vi "calcolo rendimento.vi"(0 "Array prove":refnum<vi>[](array[refnum]), 1 "DETERMINAZIONE DEL RENDIMENTO Item Names":string[][](array[string]), 2 "Dati prove":T1, 3 "TABELLE":i16[](array[numeric]), 5 "error in":errorcluster) -> (9 "Eq termico ko":bool, 10 "Coeff correlaz":dbl, 11 "Resistenze ko":bool, 14 "ripeti prova?":bool, 15 "DETERMINAZIONE DEL RENDIMENTO":string[][](array[string]), 16 "Perdite da termica":T6, 17 "Perdite da prova a vuoto 2":T2, 18 "Calcoli da step carichi":T5, 19 "error out":errorcluster)   [LabVIEW 2019]
uses:
  TypeDef/Dati collaudo.ctl
panel:
  in  "Tab Control":T3(tab)
  out "Tabella prova a freddo":i32(listbox)
  in  "Tab Control 3":enum32{"TABELLA ACQUISIZIONI", "Resistenze"}(tab)
  out "Tabella prova a vuoto":i32(listbox)
  out "Resistenze iniziali a vuoto":i32(listbox)
  out "Resistenze finali a vuoto":i32(listbox)
  in  "Tab Control 5":enum32{"TABELLA ACQUISIZIONI", "Resistenze"}(tab)
  out "Tabella prova a carico":i32(listbox)
  out "resistenze iniz a carico":i32(listbox) caption="Resistenze iniziali"
  out "resistenze fin a carico":i32(listbox) caption="Resistenze finali"
  in  "Tab Control 6":T4(tab)
  out "Tabella a freddo - termica":i32(listbox) caption="Tabella misura resistenze a freddo"
  out "Tabella riscaldamento termica":i32(listbox)
  out "Dati riscaldamento":i32(listbox)
  out "Tabella prova a rot blocc":i32(listbox)
  out "Tabella prova coppia max dati":i32(listbox)
  out "Tabella riga coppia max":i32(listbox)
  out "Tabella prova caratt mecc":i32(listbox)
  out "DETERMINAZIONE DEL RENDIMENTO":i32[](listbox)
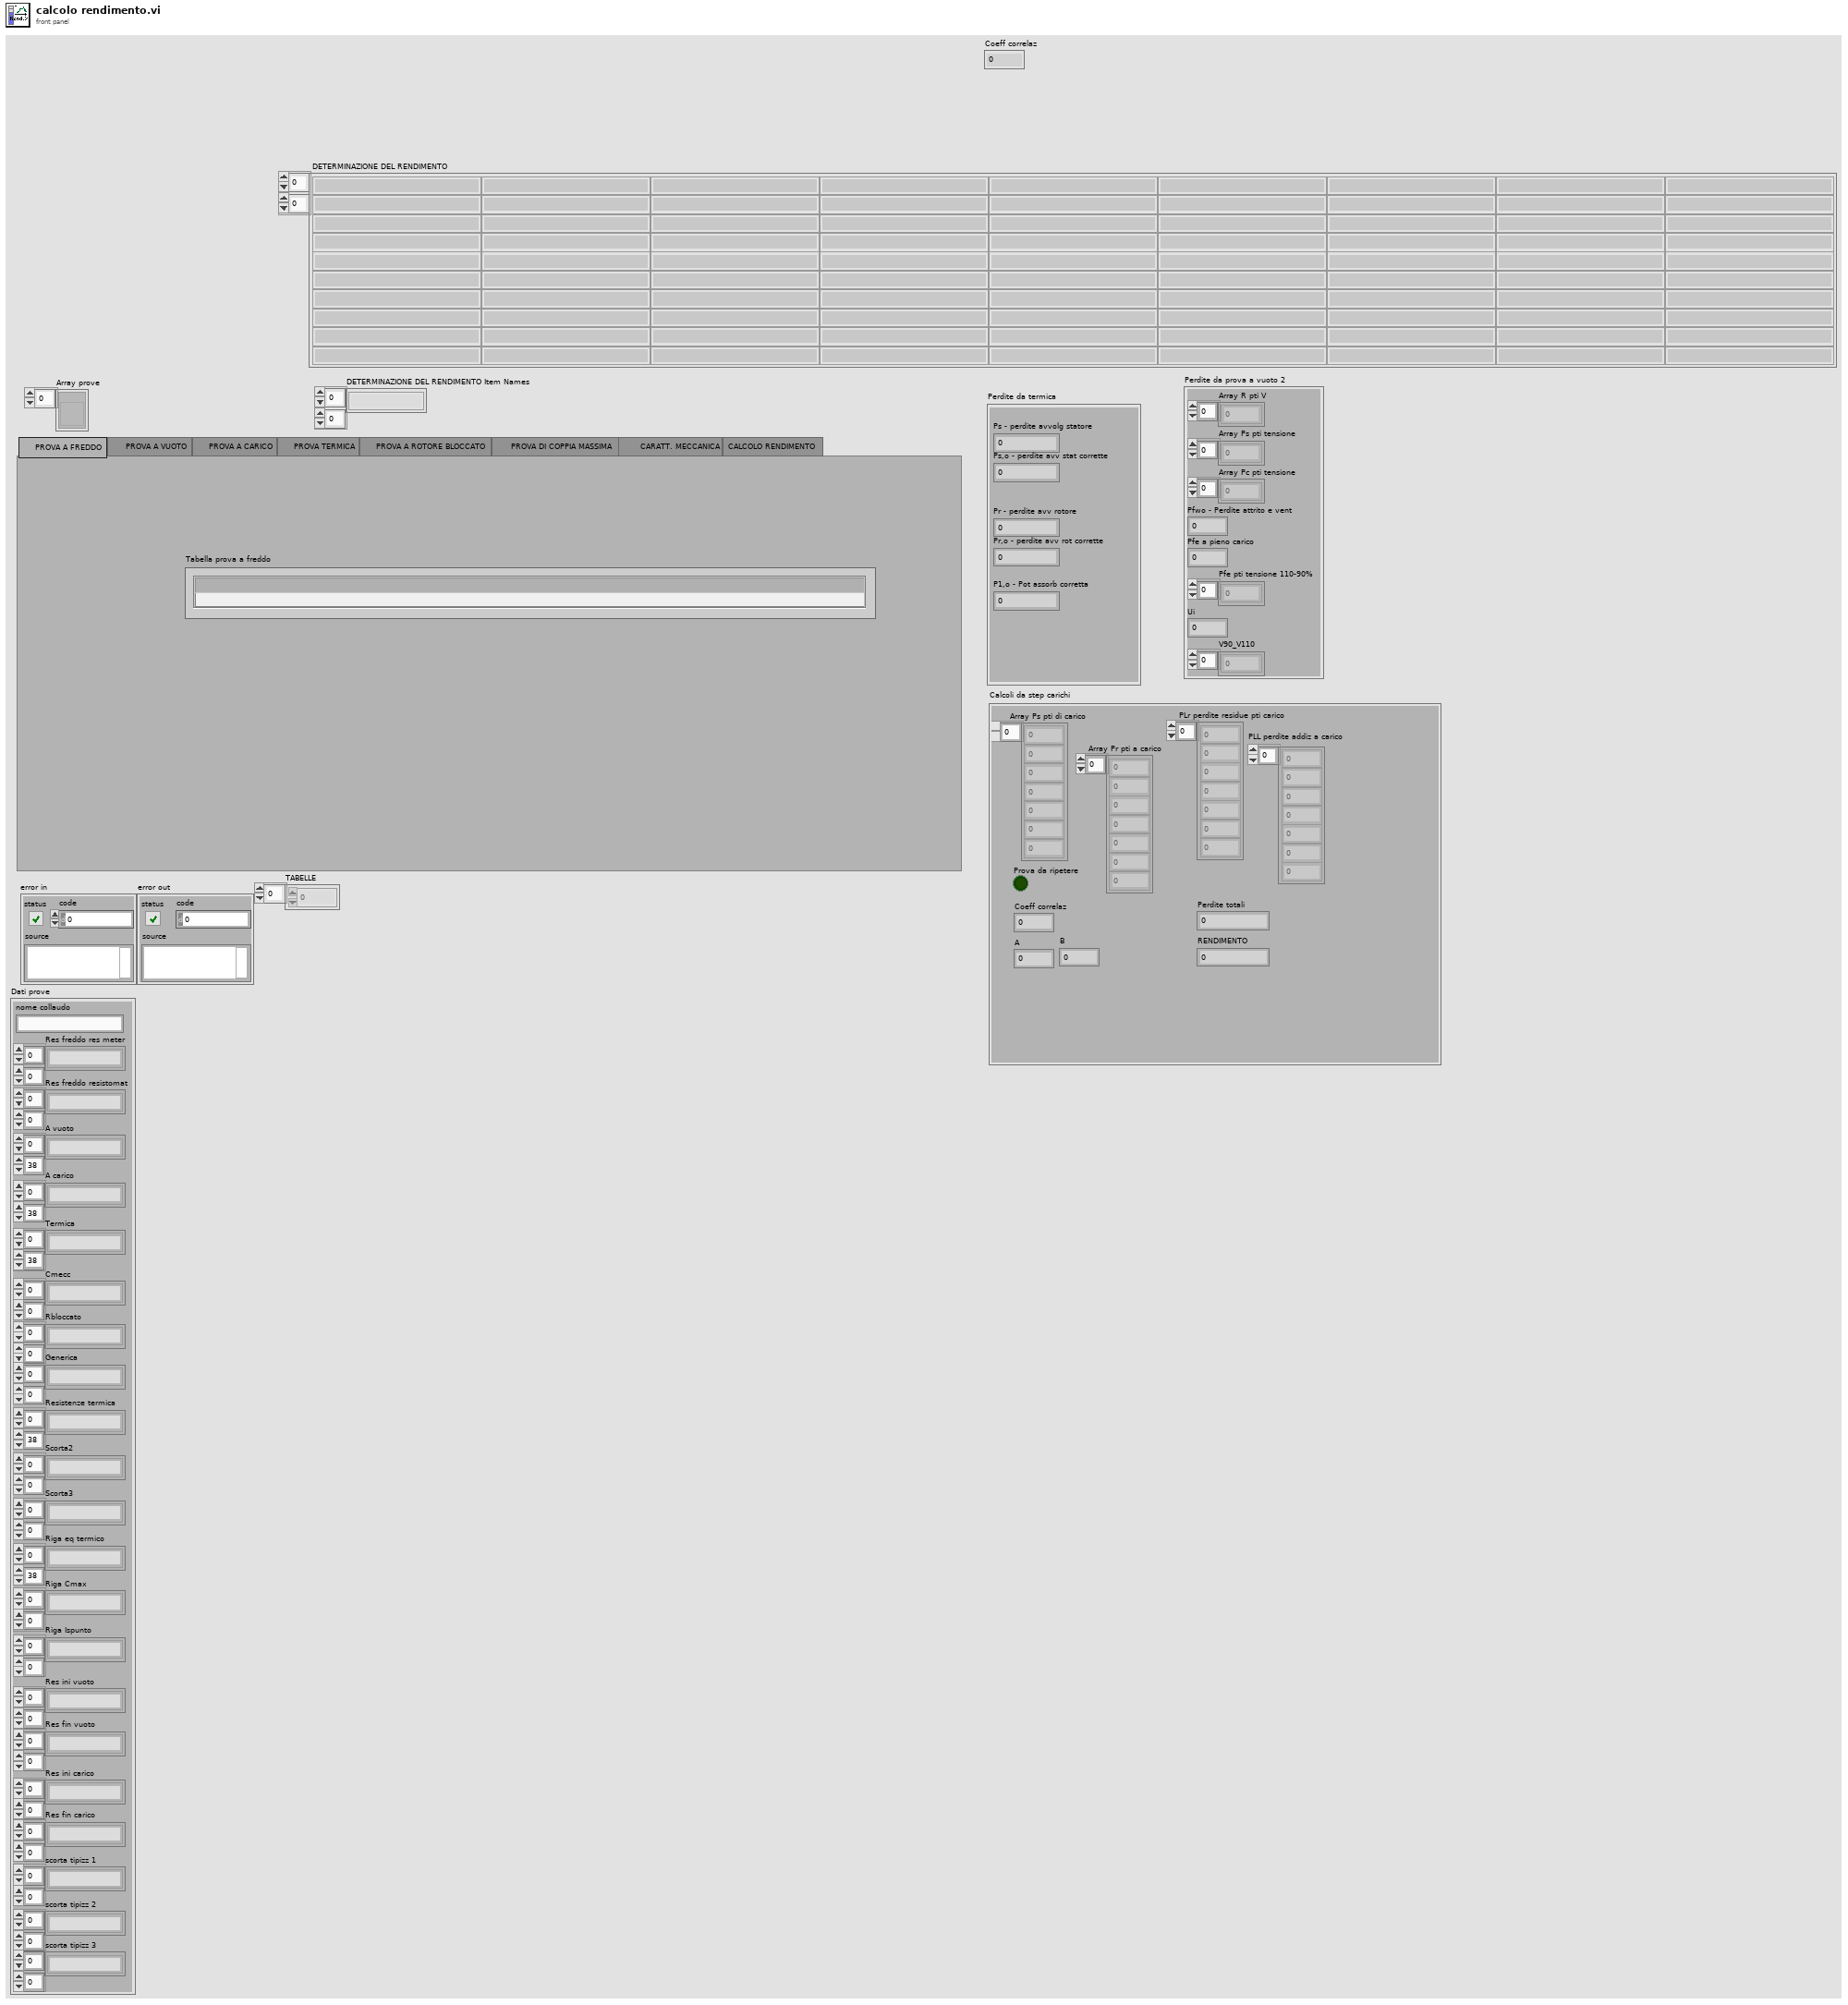
[diagram p1: front panel]
types:
  T1 = typedef "Dati collaudo.ctl" = cluster{"nome collaudo":string, "Res freddo res meter":string[][], "Res freddo resistomat":string[][], "A vuoto":string[][], "A carico":string[][], "Termica":string[][], "Cmecc":string[][], "Rbloccato":string[][], "Generica":string[][], "Resistenze termica":string[][], "Scorta2":string[][], "Scorta3":string[][], "Riga eq termico":string[][], "Riga Cmax":string[][], "Riga Ispunto":string[][], "Res ini vuoto":string[][], "Res fin vuoto":string[][], "Res ini carico":string[][], "Res fin carico":string[][], "scorta tipizz 1":string[][], "scorta tipizz 2":string[][], "scorta tipizz 3":string[][]}
  T2 = cluster{"Array R pti V":dbl[], "Array Ps pti tensione":dbl[], "Array Pc pti tensione":dbl[], "Pfwo - Perdite attrito e vent":dbl, "Pfe a pieno carico":dbl, "Pfe pti tensione 110-90% ":dbl[], "Ui":dbl, "V90_V110":dbl[]}
  T3 = enum32{"    PROVA A FREDDO", "     PROVA A VUOTO", "    PROVA A CARICO", "    PROVA TERMICA", "    PROVA A ROTORE BLOCCATO", "     PROVA DI COPPIA MASSIMA", "      CARATT. MECCANICA", "CALCOLO RENDIMENTO"}
  T4 = enum32{"DATI A FREDDO", "TABELLA ACQ. RISCALDAMENTO", "TABELLA DATI RESISTENZE - DELTA T"}
  T5 = cluster{"Array Ps pti di carico":dbl[], "Array Pr pti a carico":dbl[], "PLr perdite residue pti carico":dbl[], "A":dbl, "B":dbl, "Coeff correlaz":dbl, "Prova da ripetere":bool, "PLL perdite addiz a carico":dbl[], "Perdite totali":dbl, "RENDIMENTO":dbl}
  T6 = cluster{"Ps - perdite avvolg statore":dbl, "Ps,o - perdite avv stat corrette":dbl, "Pr - perdite avv rotore":dbl, "Pr,o - perdite avv rot corrette":dbl, "P1,o - Pot assorb corretta":dbl}
  T7 = cluster{"INDEX R eq termico":i32, "index Tamb caldo":i32, "index dt":i32}
  T8 = cluster{"INDEX P1":i32, "INDEX COPPIA":i32, "INDEX I":i32, "INDEX V":i32, "INDEX SCORR":i32, "INDEX t fluido ingresso":i32, "INDEX P resa":i32, "INDEX tempo":i32, "INDEX dt":i32}
  T9 = cluster{"INDEX P1 W":i32, "INDEX COPPIA":i32, "INDEX I":i32, "INDEX V":i32, "INDEX SCORR":i32, "INDEX t fluido ingresso":i32, "INDEX P resa W":i32, "INDEX tempo s":i32, "INDEX dt":i32}
  T10 = cluster{"INDEX P1":i32, "INDEX COPPIA":i32, "INDEX I":i32, "INDEX V":i32, "INDEX SCORR":i32, "INDEX t fluido ingresso":i32, "INDEX P resa":i32, "INDEX tempo":i32, "INDEX dt":i32}[]
  T11 = cluster{"INDEX R eq termico":i32, "index Tamb caldo":i32, "index dt":i32}[]
  T12 = cluster{"R iniz carico":dbl, "R fin carico":dbl, "Array V carico":dbl[], "Array I carico":dbl[], "Array P elett carico":dbl[], "Array Scorr carico":dbl[], "Array Presa carico":dbl[], "Array Coppia carico":dbl[]}
  T13 = cluster{"R iniz vuoto":dbl, "R fin vuoto":dbl, "Array V0 a vuoto":dbl[], "Array I0 a vuoto":dbl[], "Array P0 a vuoto":dbl[], "Array Scorr a vuoto":dbl[]}
  T14 = cluster{"P1elettrica":dbl, "Coppia":dbl, "I corrente":dbl, "U tensione":dbl, "RPM":dbl, "Freq":dbl, "R eq termico":dbl, "Scorrimento":dbl}
  T15 = cluster{"Rendimenti % a carico":dbl[], "P1 corretta":dbl[], "Scorr corretto":dbl[], "Perdite nel ferro":dbl[], "Perdite mecc corrette":dbl[], "Perdite addiz":dbl[], "perdite statore corrette":dbl[], "perdite rotore corrette":dbl[]}
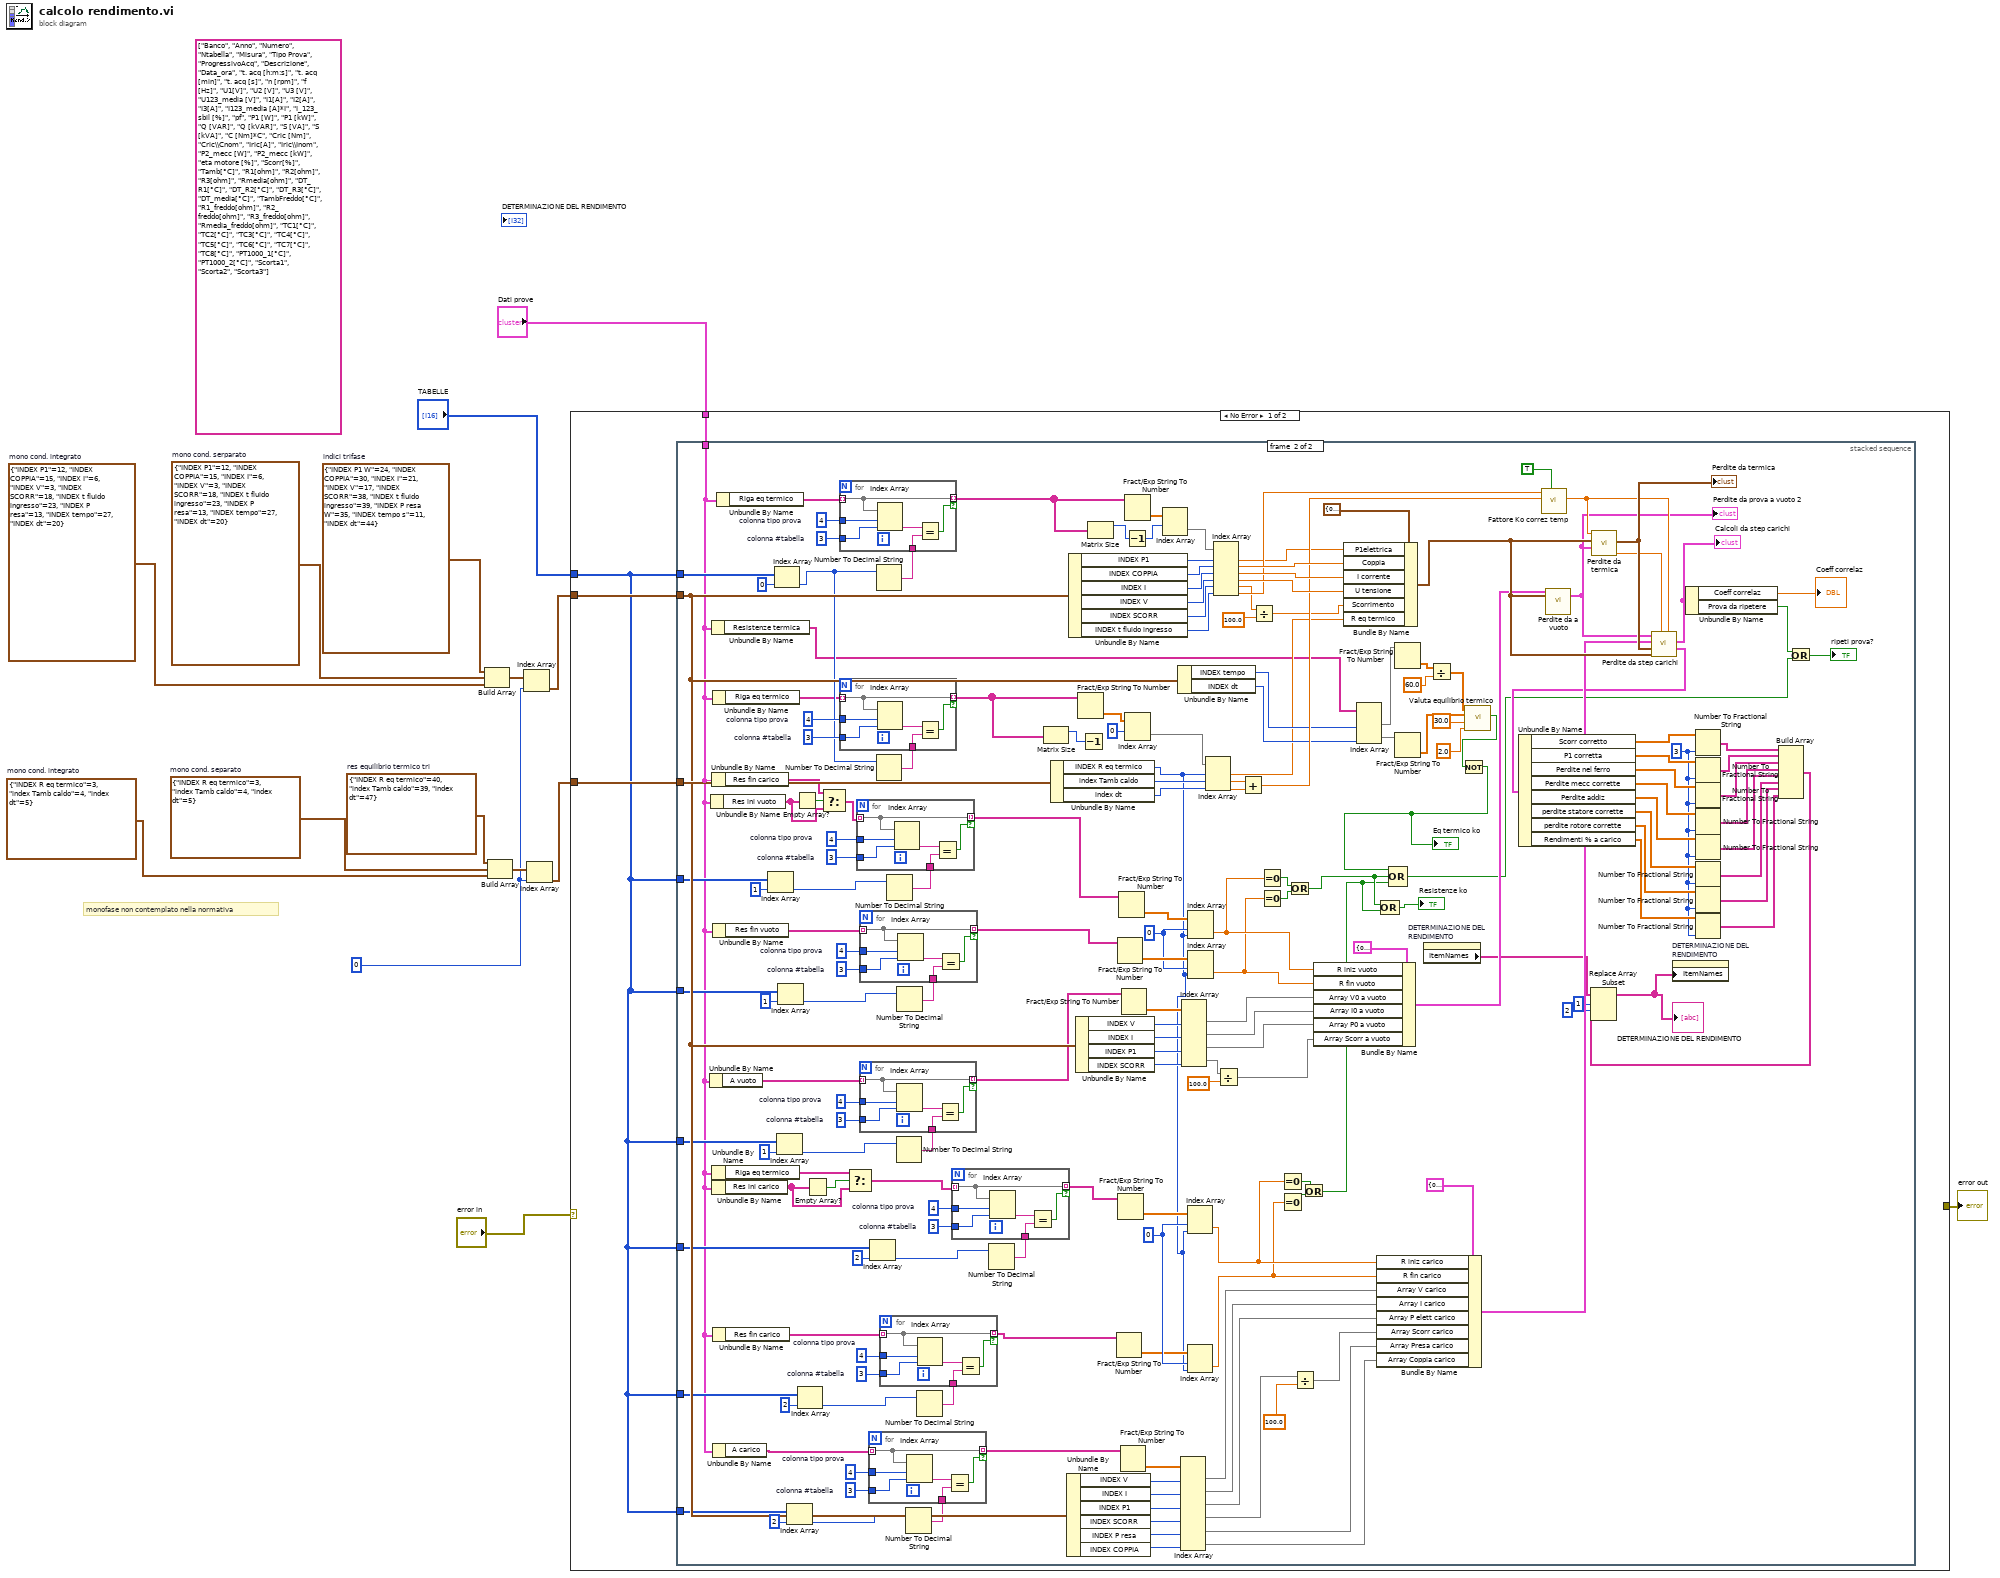
[diagram p0: block diagram]
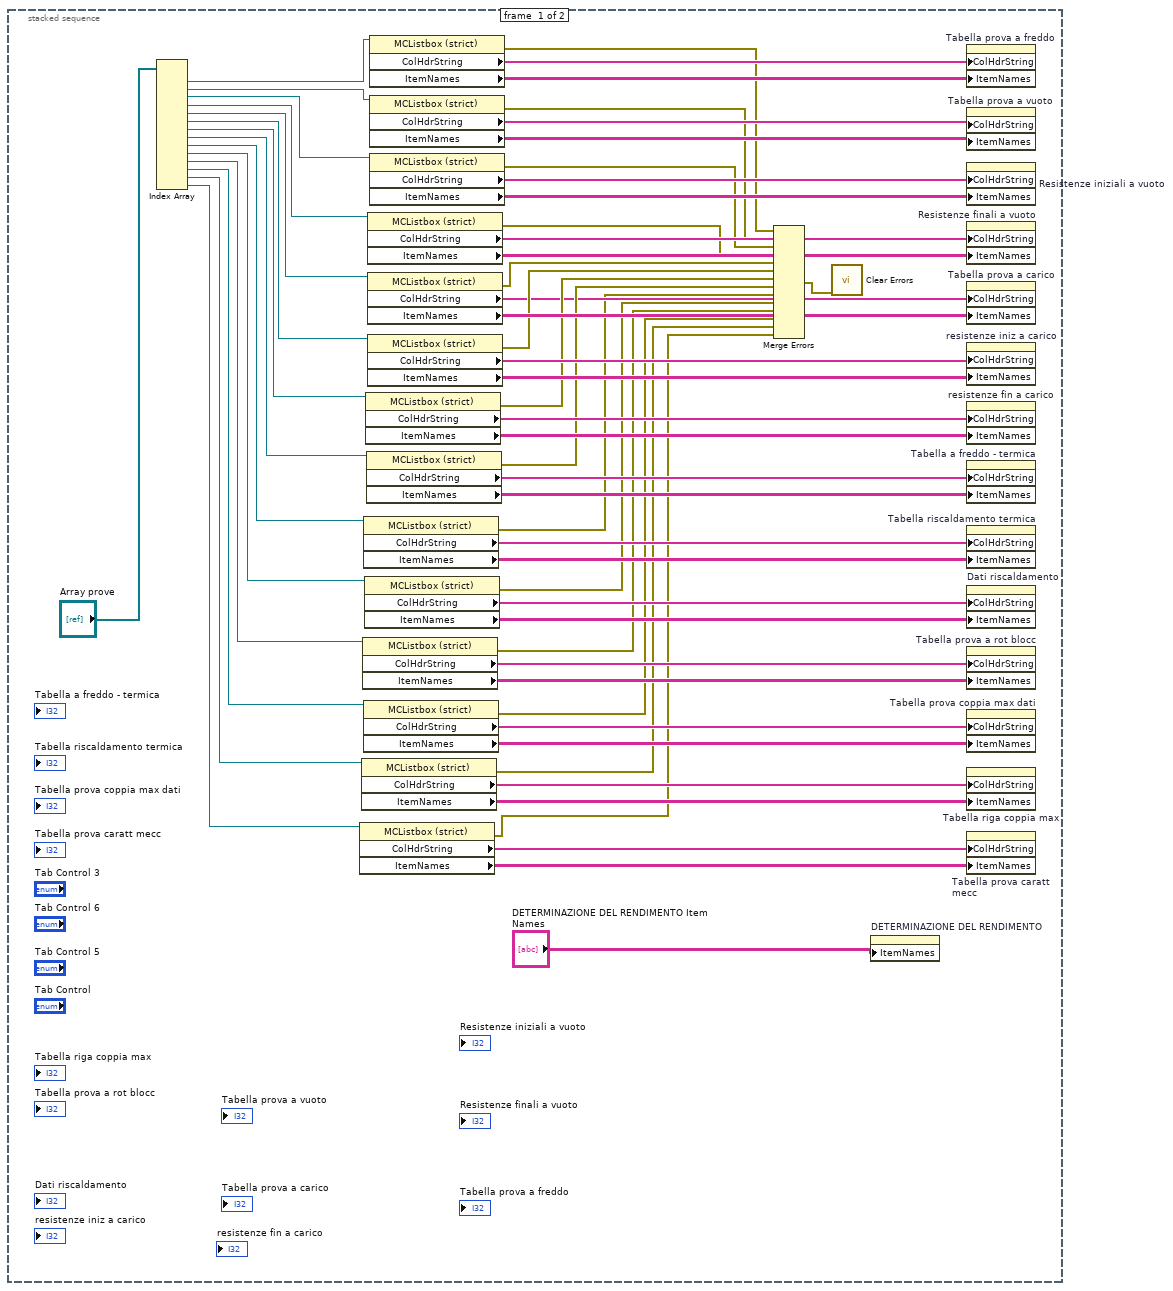
[diagram p2: hidden frame]
diagram:
  (unwired) string[] ["Banco", "Anno", "Numero", "Ntabella", "Misura", "Tipo Prova", "ProgressivoAcq", "Descrizione", "Data_ora", "t. acq [h:m:s]", "t. acq [min]", "t. acq [s]", "n [rpm]", "f [Hz]", "U1[V]", "U2 [V]", "U3 [V]", "U123_media [V]", "I1[A]", "I2[A]", "I3[A]", "I123_media [A]*I", "I_123_sbil [%]", "pf", "P1 [W]", "P1 [kW]", "Q [VAR]", "Q [kVAR]", "S [VA]", "S [kVA]", "C [Nm]*C", "Cric [Nm]", "Cric\\Cnom", "Iric[A]", "Iric\\Inom", "P2_mecc [W]", "P2_mecc [kW]", "eta motore [%]", "Scorr[%]", "Tamb[°C]", "R1[ohm]", "R2[ohm]", "R3[ohm]", "Rmedia[ohm]", "DT_R1[°C]", "DT_R2[°C]", "DT_R3[°C]", "DT_media[°C]", "TambFreddo[°C]", "R1_freddo[ohm]", "R2_freddo[ohm]", "R3_freddo[ohm]", "Rmedia_freddo[ohm]", "TC1[°C]", "TC2[°C]", "TC3[°C]", "TC4[°C]", "TC5[°C]", "TC6[°C]", "TC7[°C]", "TC8[°C]", "PT1000_1[°C]", "PT1000_2[°C]", "Scorta1", "Scorta2", "Scorta3"] ("ETICHETTE")
  w3 = 0 ("index")
  w6 = T7 {"INDEX R eq termico"=3, "index Tamb caldo"=4, "index dt"=5}  # mono cond. integrato
  w12 = T8 {"INDEX P1"=12, "INDEX COPPIA"=15, "INDEX I"=6, "INDEX V"=3, "INDEX SCORR"=18, "INDEX t fluido ingresso"=23, "INDEX P resa"=13, "INDEX tempo"=27, "INDEX dt"=20}  # mono cond. integrato
  w7 = T7 {"INDEX R eq termico"=3, "index Tamb caldo"=4, "index dt"=5}  # mono cond. separato
  w13 = T8 {"INDEX P1"=12, "INDEX COPPIA"=15, "INDEX I"=6, "INDEX V"=3, "INDEX SCORR"=18, "INDEX t fluido ingresso"=23, "INDEX P resa"=13, "INDEX tempo"=27, "INDEX dt"=20}  # mono cond. serparato
  w8 = T7 {"INDEX R eq termico"=40, "index Tamb caldo"=39, "index dt"=47}  # res equilibrio termico tri
  w10 = T9 {"INDEX P1 W"=24, "INDEX COPPIA"=30, "INDEX I"=21, "INDEX V"=17, "INDEX SCORR"=38, "INDEX t fluido ingresso"=39, "INDEX P resa W"=35, "INDEX tempo s"=11, "INDEX dt"=44}  # indici trifase
  # "monofase non contemplato nella normativa"
  n1 = Build Array(w10, w13, w12) -> (w11:T10)
  n2 = Build Array(w8, w7, w6) -> (w5:T11)
  n3 = Index Array(array=w11, index=w3) -> (element=w9:T8)
  n4 = Index Array(array=w5, index=w3) -> (element=w4:T7)
  n5 = case shown="No Error" "error in" {
    selector: "error in" -> [_ w321]
    tunnel: [_ w321] -> w14
    tunnel: w9 -> [w19 _]
    tunnel: w4 -> [w18 _]
    tunnel: "Dati prove" -> [w17 _]
    tunnel: "TABELLE" -> [w16 _]
    frame No Error {
      n6 = stacked-sequence {
        tunnel: w19 -> [_ w158]
        tunnel: w18 -> [_ w161]
        tunnel: w17 -> [_ w82]
        tunnel: w16 -> [_ w144]
        tunnel: w16 -> [_ w118]
        tunnel: w16 -> [_ w110]
        tunnel: w16 -> [_ w109]
        tunnel: w16 -> [_ w108]
        tunnel: w16 -> [_ w100]
        tunnel: w16 -> [_ w92]
        frame #0 {
          n7 = Index Array(array="Array prove") -> (element #1=w76:refnum<vi>, element #2=w73:refnum<vi>, element #3=w70:refnum<vi>, element #4=w67:refnum<vi>, element #5=w64:refnum<vi>, element #6=w62:refnum<vi>, element #7=w59:refnum<vi>, element #8=w56:refnum<vi>, element #9=w53:refnum<vi>, element #10=w50:refnum<vi>, element #11=w47:refnum<vi>, element #12=w44:refnum<vi>, element #13=w41:refnum<vi>, element #14=w38:refnum<vi>)  [unwired: 14 in]
          n8 = property class="MCListbox (strict)"(reference=w38) -> (error out=w21:errorcluster, "ColHdrString"=w37:string[], "ItemNames"=w36:string[][])  [unwired: 1 in, 1 out]
          n9 = property class="MCListbox (strict)"(reference=w41) -> (error out=w22:errorcluster, "ColHdrString"=w40:string[], "ItemNames"=w39:string[][])  [unwired: 1 in, 1 out]
          n10 = property class="MCListbox (strict)"(reference=w47) -> (error out=w24:errorcluster, "ColHdrString"=w46:string[], "ItemNames"=w45:string[][])  [unwired: 1 in, 1 out]
          n11 = property class="MCListbox (strict)"(reference=w53) -> (error out=w26:errorcluster, "ColHdrString"=w52:string[], "ItemNames"=w51:string[][])  [unwired: 1 in, 1 out]
          n12 = property class="MCListbox (strict)"(reference=w44) -> (error out=w23:errorcluster, "ColHdrString"=w43:string[], "ItemNames"=w42:string[][])  [unwired: 1 in, 1 out]
          n13 = property class="MCListbox (strict)"(reference=w50) -> (error out=w25:errorcluster, "ColHdrString"=w49:string[], "ItemNames"=w48:string[][])  [unwired: 1 in, 1 out]
          n14 = property class="MCListbox (strict)"(reference=w59) -> (error out=w29:errorcluster, "ColHdrString"=w58:string[], "ItemNames"=w57:string[][])  [unwired: 1 in, 1 out]
          n15 = property class="MCListbox (strict)"(reference=w56) -> (error out=w28:errorcluster, "ColHdrString"=w55:string[], "ItemNames"=w54:string[][])  [unwired: 1 in, 1 out]
          n16 = property class="MCListbox (strict)"(reference=w67) -> (error out=w32:errorcluster, "ColHdrString"=w66:string[], "ItemNames"=w65:string[][])  [unwired: 1 in, 1 out]
          n17 = property class="MCListbox (strict)"(reference=w64) -> (error out=w31:errorcluster, "ColHdrString"=w27:string[], "ItemNames"=w63:string[][])  [unwired: 1 in, 1 out]
          n18 = property class="MCListbox (strict)"(reference=w62) -> (error out=w30:errorcluster, "ColHdrString"=w61:string[], "ItemNames"=w60:string[][])  [unwired: 1 in, 1 out]
          n19 = property class="MCListbox (strict)"(reference=w76) -> (error out=w35:errorcluster, "ColHdrString"=w75:string[], "ItemNames"=w74:string[][])  [unwired: 1 in, 1 out]
          n20 = property class="MCListbox (strict)"(reference=w73) -> (error out=w34:errorcluster, "ColHdrString"=w72:string[], "ItemNames"=w71:string[][])  [unwired: 1 in, 1 out]
          n21 = property class="MCListbox (strict)"(reference=w70) -> (error out=w33:errorcluster, "ColHdrString"=w69:string[], "ItemNames"=w68:string[][])  [unwired: 1 in, 1 out]
          n22 = Merge Errors(w35, w34, w33, w32, w31, w30, w29, w28, w26, w25, w24, w23, w22, w21) -> (w20:errorcluster)
          n23 = call <vilib>:"Clear Errors.vi"("error in (no error)"=w20) -> ()  [unwired: 5 in, 2 out]
          n24 = property on="DETERMINAZIONE DEL RENDIMENTO" class="MCListbox (strict)"("ItemNames"="DETERMINAZIONE DEL RENDIMENTO Item Names") -> ()  [unwired: 2 in, 2 out]
          n25 = property on="Tabella prova a freddo" class="MCListbox (strict)"("ColHdrString"=w75, "ItemNames"=w74) -> ()  [unwired: 2 in, 2 out]
          n26 = property on="Tabella prova a vuoto" class="MCListbox (strict)"("ColHdrString"=w72, "ItemNames"=w71) -> ()  [unwired: 2 in, 2 out]
          n27 = property on="Resistenze iniziali a vuoto" class="MCListbox (strict)"("ColHdrString"=w69, "ItemNames"=w68) -> ()  [unwired: 2 in, 2 out]
          n28 = property on="Resistenze finali a vuoto" class="MCListbox (strict)"("ColHdrString"=w66, "ItemNames"=w65) -> ()  [unwired: 2 in, 2 out]
          n29 = property on="Tabella prova a carico" class="MCListbox (strict)"("ColHdrString"=w27, "ItemNames"=w63) -> ()  [unwired: 2 in, 2 out]
          n30 = property on="resistenze iniz a carico" class="MCListbox (strict)"("ColHdrString"=w61, "ItemNames"=w60) -> ()  [unwired: 2 in, 2 out]
          n31 = property on="resistenze fin a carico" class="MCListbox (strict)"("ColHdrString"=w58, "ItemNames"=w57) -> ()  [unwired: 2 in, 2 out]
          n32 = property on="Tabella a freddo - termica" class="MCListbox (strict)"("ColHdrString"=w55, "ItemNames"=w54) -> ()  [unwired: 2 in, 2 out]
          n33 = property on="Tabella riscaldamento termica" class="MCListbox (strict)"("ColHdrString"=w52, "ItemNames"=w51) -> ()  [unwired: 2 in, 2 out]
          n34 = property on="Dati riscaldamento" class="MCListbox (strict)"("ColHdrString"=w49, "ItemNames"=w48) -> ()  [unwired: 2 in, 2 out]
          n35 = property on="Tabella prova a rot blocc" class="MCListbox (strict)"("ColHdrString"=w46, "ItemNames"=w45) -> ()  [unwired: 2 in, 2 out]
          n36 = property on="Tabella prova coppia max dati" class="MCListbox (strict)"("ColHdrString"=w43, "ItemNames"=w42) -> ()  [unwired: 2 in, 2 out]
          n37 = property on="Tabella riga coppia max" class="MCListbox (strict)"("ColHdrString"=w40, "ItemNames"=w39) -> ()  [unwired: 2 in, 2 out]
          n38 = property on="Tabella prova caratt mecc" class="MCListbox (strict)"("ColHdrString"=w37, "ItemNames"=w36) -> ()  [unwired: 2 in, 2 out]
        }
        frame #1 {
          w96 = 3  # colonna #tabella
          w95 = 4  # colonna tipo prova
          w106 = 3  # colonna #tabella
          w107 = 4  # colonna tipo prova
          w113 = 3  # colonna #tabella
          w112 = 4  # colonna tipo prova
          w123 = 3  # colonna #tabella
          w124 = 4  # colonna tipo prova
          w128 = 3  # colonna #tabella
          w127 = 4  # colonna tipo prova
          w136 = 3  # colonna #tabella
          w137 = 4  # colonna tipo prova
          w141 = 3  # colonna #tabella
          w140 = 4  # colonna tipo prova
          w148 = 3  # colonna #tabella
          w149 = 4  # colonna tipo prova
          w209 = i16 3 ("precision (6)")
          w248 = 0 ("index (row)")
          w254 = 0 ("index (row)")
          n39 = Unbundle By Name(w82) -> ("A vuoto"=w120:string[][])
          n40 = Unbundle By Name(w82) -> ("Res ini vuoto"=w86:string[][])
          n41 = Unbundle By Name(w82) -> ("Resistenze termica"=w81:string[][])
          n42 = Unbundle By Name(w82) -> ("Res fin carico"=w83:string[][])
          n43 = Unbundle By Name(w82) -> ("Riga eq termico"=w90:string[][])
          n44 = Unbundle By Name(w82) -> ("Res ini carico"=w88:string[][])
          n45 = Unbundle By Name(w82) -> ("Riga eq termico"=w84:string[][])
          n46 = Unbundle By Name(w82) -> ("Res fin vuoto"=w126:string[][])
          n47 = Unbundle By Name(w82) -> ("Res fin carico"=w102:string[][])
          n48 = Unbundle By Name(w82) -> ("A carico"=w94:string[][])
          n49 = Unbundle By Name(w82) -> ("Riga eq termico"=w147:string[][])
          n50 = Index Array(array=w118, index=1) -> (element=w132:i16)
          n51 = Index Array(array=w144, index=0) -> (element=w138:i16)
          n52 = Index Array(array=w109, index=1) -> (element=w121:i16)
          n53 = Index Array(array=w110, index=1) -> (element=w131:i16)
          n54 = Index Array(array=w92, index=2) -> (element=w98:i16)
          n55 = Empty Array?(array=w86) -> (empty?=w87:bool)
          n56 = Index Array(array=w100, index=2) -> (element=w104:i16)
          n57 = Empty Array?(array=w88) -> (empty?=w91:bool)
          n58 = Select(t=w83, s=w87, f=w86) -> (s? t:f=w85:string[][])
          n59 = Select(t=w90, s=w91, f=w88) -> (s? t:f=w89:string[][])
          n60 = Index Array(array=w108, index=2) -> (element=w115:i16)
          n61 = Number To Decimal String(number=w138) -> (decimal integer string=w146:string)  [unwired: 1 in]
          n62 = for {
            tunnel: w147 -> [w319] mode=indexing
            tunnel: [w319] -> w145 mode=indexing if=w315
            tunnel: w149 -> [w320]
            tunnel: w148 -> [w318]
            tunnel: w146 -> [w316]
            n63 = Index Array(array=w319, index #1=w320, index #2=w318) -> (element #2=w317:string)  [unwired: 1 out]
            n64 = Equal?(x=w317, y=w316) -> (x = y?=w315:bool)
          }
          n65 = Number To Decimal String(number=w138) -> (decimal integer string=w142:string)  [unwired: 1 in]
          n66 = for {
            tunnel: w84 -> [w313] mode=indexing
            tunnel: [w313] -> w139 mode=indexing if=w309
            tunnel: w140 -> [w314]
            tunnel: w141 -> [w312]
            tunnel: w142 -> [w310]
            n67 = Index Array(array=w313, index #1=w314, index #2=w312) -> (element #2=w311:string)  [unwired: 1 out]
            n68 = Equal?(x=w311, y=w310) -> (x = y?=w309:bool)
          }
          n69 = Number To Decimal String(number=w132) -> (decimal integer string=w135:string)  [unwired: 1 in]
          n70 = for {
            tunnel: w85 -> [w307] mode=indexing
            tunnel: [w307] -> w134 mode=indexing if=w303
            tunnel: w137 -> [w308]
            tunnel: w136 -> [w306]
            tunnel: w135 -> [w304]
            n71 = Index Array(array=w307, index #1=w308, index #2=w306) -> (element #2=w305:string)  [unwired: 1 out]
            n72 = Equal?(x=w305, y=w304) -> (x = y?=w303:bool)
          }
          n73 = Number To Decimal String(number=w121) -> (decimal integer string=w117:string)  [unwired: 1 in]
          n74 = for {
            tunnel: w120 -> [w295] mode=indexing
            tunnel: [w295] -> w119 mode=indexing if=w291
            tunnel: w124 -> [w296]
            tunnel: w123 -> [w294]
            tunnel: w117 -> [w292]
            n75 = Index Array(array=w295, index #1=w296, index #2=w294) -> (element #2=w293:string)  [unwired: 1 out]
            n76 = Equal?(x=w293, y=w292) -> (x = y?=w291:bool)
          }
          n77 = Number To Decimal String(number=w131) -> (decimal integer string=w129:string)  [unwired: 1 in]
          n78 = for {
            tunnel: w126 -> [w301] mode=indexing
            tunnel: [w301] -> w125 mode=indexing if=w297
            tunnel: w127 -> [w302]
            tunnel: w128 -> [w300]
            tunnel: w129 -> [w298]
            n79 = Index Array(array=w301, index #1=w302, index #2=w300) -> (element #2=w299:string)  [unwired: 1 out]
            n80 = Equal?(x=w299, y=w298) -> (x = y?=w297:bool)
          }
          n81 = Number To Decimal String(number=w98) -> (decimal integer string=w99:string)  [unwired: 1 in]
          n82 = for {
            tunnel: w94 -> [w277] mode=indexing
            tunnel: [w277] -> w93 mode=indexing if=w273
            tunnel: w95 -> [w278]
            tunnel: w96 -> [w276]
            tunnel: w99 -> [w274]
            n83 = Index Array(array=w277, index #1=w278, index #2=w276) -> (element #2=w275:string)  [unwired: 1 out]
            n84 = Equal?(x=w275, y=w274) -> (x = y?=w273:bool)
          }
          n85 = Number To Decimal String(number=w104) -> (decimal integer string=w103:string)  [unwired: 1 in]
          n86 = for {
            tunnel: w102 -> [w283] mode=indexing
            tunnel: [w283] -> w101 mode=indexing if=w279
            tunnel: w107 -> [w284]
            tunnel: w106 -> [w282]
            tunnel: w103 -> [w280]
            n87 = Index Array(array=w283, index #1=w284, index #2=w282) -> (element #2=w281:string)  [unwired: 1 out]
            n88 = Equal?(x=w281, y=w280) -> (x = y?=w279:bool)
          }
          n89 = Number To Decimal String(number=w115) -> (decimal integer string=w116:string)  [unwired: 1 in]
          n90 = for {
            tunnel: w89 -> [w289] mode=indexing
            tunnel: [w289] -> w111 mode=indexing if=w285
            tunnel: w112 -> [w290]
            tunnel: w113 -> [w288]
            tunnel: w116 -> [w286]
            n91 = Index Array(array=w289, index #1=w290, index #2=w288) -> (element #2=w287:string)  [unwired: 1 out]
            n92 = Equal?(x=w287, y=w286) -> (x = y?=w285:bool)
          }
          n93 = Matrix Size(0:w139) -> (1:w239:i32)  [unwired: 1 out]
          n94 = Unbundle By Name(w161) -> ("INDEX R eq termico"=w80:i32, "index Tamb caldo"=w160:i32, "index dt"=w159:i32)
          n95 = Unbundle By Name(w158) -> ("INDEX V"=w167:i32, "INDEX I"=w166:i32, "INDEX P1"=w165:i32, "INDEX SCORR"=w164:i32, "INDEX P resa"=w163:i32, "INDEX COPPIA"=w162:i32)
          n96 = Unbundle By Name(w158) -> ("INDEX P1"=w177:i32, "INDEX COPPIA"=w176:i32, "INDEX I"=w175:i32, "INDEX V"=w174:i32, "INDEX SCORR"=w173:i32, "INDEX t fluido ingresso"=w172:i32)
          n97 = Unbundle By Name(w158) -> ("INDEX V"=w171:i32, "INDEX I"=w170:i32, "INDEX P1"=w169:i32, "INDEX SCORR"=w168:i32)
          n98 = Fract/Exp String To Number(string=w139) -> (number=w264:dbl[][])  [unwired: 3 in, 1 out]
          n99 = Decrement(x=w239) -> ()  [unwired: 1 out]
          n100 = Matrix Size(0:w145) -> (1:w241:i32)  [unwired: 1 out]
          n101 = Fract/Exp String To Number(string=w101) -> (number=w247:dbl[][])  [unwired: 3 in, 1 out]
          n102 = Fract/Exp String To Number(string=w125) -> (number=w255:dbl[][])  [unwired: 3 in, 1 out]
          n103 = Fract/Exp String To Number(string=w111) -> (number=w246:dbl[][])  [unwired: 3 in, 1 out]
          n104 = Fract/Exp String To Number(string=w134) -> (number=w256:dbl[][])  [unwired: 3 in, 1 out]
          n105 = Fract/Exp String To Number(string=w93) -> (number=w249:dbl[][])  [unwired: 3 in, 1 out]
          n106 = Fract/Exp String To Number(string=w119) -> (number=w253:dbl[][])  [unwired: 3 in, 1 out]
          n107 = Fract/Exp String To Number(string=w145) -> (number=w269:dbl[][])  [unwired: 3 in, 1 out]
          n108 = Decrement(x=w241) -> (x-1=w240:i32)
          n109 = Index Array(array=w264, index (row)=0) -> (element=w261:dbl[])  [unwired: 1 in]
          n110 = Index Array(array=w269, index (row)=w240) -> (element=w268:dbl[])  [unwired: 1 in]
          n111 = Unbundle By Name(w158) -> ("INDEX tempo"=w157:i32, "INDEX dt"=w156:i32)
          n112 = Index Array(array=w249, index (col) #1=w167, index (col) #2=w166, index (col) #3=w165, index (col) #4=w164, index (col) #5=w163, index (col) #6=w162) -> (element #1=w245:dbl[], element #2=w244:dbl[], element #3=w182:dbl[], element #4=w235:dbl[], element #5=w183:dbl[], element #6=w231:dbl[])  [unwired: 6 in]
          n113 = Index Array(array=w253, index (col) #1=w171, index (col) #2=w170, index (col) #3=w169, index (col) #4=w168) -> (element #1=w252:dbl[], element #2=w251:dbl[], element #3=w184:dbl[], element #4=w238:dbl[])  [unwired: 4 in]
          n114 = Index Array(array=w246, index (row)=w248, index (col)=w80) -> (element=w188:dbl)
          n115 = Index Array(array=w247, index (row)=w248, index (col)=w80) -> (element=w187:dbl)
          n116 = Index Array(array=w256, index (row)=w254, index (col)=w80) -> (element=w198:dbl)
          n117 = Index Array(array=w255, index (row)=w254, index (col)=w80) -> (element=w197:dbl)
          n118 = Index Array(array=w261, index #1=w80, index #2=w160, index #3=w159) -> (element #1=w151:dbl, element #2=w260:dbl, element #3=w259:dbl)
          n119 = Index Array(array=w268, index #1=w177, index #2=w176, index #3=w175, index #4=w174, index #5=w173, index #6=w172) -> (element #1=w185:dbl, element #2=w267:dbl, element #3=w266:dbl, element #4=w265:dbl, element #5=w232:dbl, element #6=w262:dbl)
          n120 = Divide(x=w238, y=100.0 ("x+y")) -> (x/y=w153:dbl[])
          n121 = Add(x=w260, y=w259) -> (x+y=w258:dbl)
          n122 = Divide(x=w232, y=100.0 ("x+y")) -> (x/y=w79:dbl)
          n123 = Equal To 0?(x=w198) -> (x = 0?=w200:bool)
          n124 = Equal To 0?(x=w197) -> (x = 0?=w201:bool)
          n125 = Equal To 0?(x=w188) -> (x = 0?=w189:bool)
          n126 = Equal To 0?(x=w187) -> (x = 0?=w190:bool)
          n127 = Or(x=w200, y=w201) -> (x .or. y?=w199:bool)
          n128 = Divide(x=w235, y=100.0 ("x+y")) -> (x/y=w234:dbl[])
          n129 = Or(x=w189, y=w190) -> (x .or. y?=w186:bool)
          n130 = Bundle By Name(cluster=T13 {"R iniz vuoto"=0.0, "R fin vuoto"=0.0, "Array V0 a vuoto"=[], "Array I0 a vuoto"=[], "Array P0 a vuoto"=[], "Array Scorr a vuoto"=[]} ("Acquisizioni vuoto"), "R iniz vuoto"=w198, "R fin vuoto"=w197, "Array V0 a vuoto"=w252, "Array I0 a vuoto"=w251, "Array P0 a vuoto"=w184, "Array Scorr a vuoto"=w153) -> (w250:T13)
          n131 = Bundle By Name(cluster=T14 {"P1elettrica"=0.0, "Coppia"=0.0, "I corrente"=0.0, "U tensione"=0.0, "RPM"=0.0, "Freq"=0.0, "R eq termico"=0.0, "Scorrimento"=0.0} ("Acqisizioni termica"), "P1elettrica"=w185, "Coppia"=w267, "I corrente"=w266, "U tensione"=w265, "Scorrimento"=w79, "R eq termico"=w151) -> (w263:T14)
          n132 = Index Array(array=w81, index (col) #1=w157, index (col) #2=w156) -> (element #1=w205:string[], element #2=w206:string[])  [unwired: 2 in]
          n133 = Bundle By Name(cluster=T12 {"R iniz carico"=0.0, "R fin carico"=0.0, "Array V carico"=[], "Array I carico"=[], "Array P elett carico"=[], "Array Scorr carico"=[], "Array Presa carico"=[], "Array Coppia carico"=[]} ("Acquisizioni step carichi"), "R iniz carico"=w188, "R fin carico"=w187, "Array V carico"=w245, "Array I carico"=w244, "Array P elett carico"=w182, "Array Scorr carico"=w234, "Array Presa carico"=w183, "Array Coppia carico"=w231) -> (w242:T12)
          n134 = Compound Arithmetic op=OR(w199, w186) -> (→"Resistenze ko":bool)
          n135 = Fract/Exp String To Number(string=w205) -> (number=w179:dbl[])  [unwired: 3 in, 1 out]
          n136 = Fract/Exp String To Number(string=w206) -> (number=w204:dbl[])  [unwired: 3 in, 1 out]
          n137 = property on="DETERMINAZIONE DEL RENDIMENTO" class="MCListbox (strict)"() -> ("ItemNames"=w211:string[][])  [unwired: 2 in, 2 out]
          n138 = Divide(x=w179, y=60.0) -> (x/y=w180:dbl[])
          n139 = call "Valuta equilibrio termico.vi"("Variazione T eqil term (°C)"=2.0, "Tempo equilibrio termico (min)"=30.0, "Array Dt"=w204, "Array Time"=w180) -> ("Equilibrio termico"=w192:bool)  [unwired: 7 in]
          n140 = Not(x=w192) -> (.not. x?=w191:bool)
          "Eq termico ko" <- w191
          n141 = Compound Arithmetic op=OR(w191, w199, w186) -> (w193:bool)
          n142 = call "Fattore Ko correz temp.vi"("Rame?"=TRUE, "T avvolg a fine prova (°C)"=w258, "T fluido ingresso (°C)"=w262) -> ("Ko"=w229:dbl)  [unwired: 8 in]
          n143 = call "Perdite da a vuoto.vi"("Acquisizioni vuoto"=w250, "Acqisizioni termica"=w263) -> ("Perdite da prova a vuoto"=w181:T2)  [unwired: 17 in]
          "Perdite da prova a vuoto 2" <- w181
          n144 = call "Perdite da termica.vi"("Perdite da prova a vuoto 2"=w181, "Acqisizioni termica"=w263, "Ko - correz temp"=w229) -> ("Scorr 0"=w230:dbl, "Perdite da termica"=w272:T6)  [unwired: 7 in]
          "Perdite da termica" <- w272
          n145 = call "Perdite da step carichi.vi"("k0"=w229, "Scorr 0"=w230, "Acqisizioni termica"=w263, "Perdite da termica"=w272, "Acquisizioni step carichi"=w242, "Perdite da prova a vuoto 2"=w181) -> ("RISULTATI"=w228:T15, "Calcoli da step carichi"=w207:T5)  [unwired: 4 in]
          "Calcoli da step carichi" <- w207
          n146 = Unbundle By Name(w228) -> ("Scorr corretto"=w227:dbl[], "P1 corretta"=w226:dbl[], "Perdite nel ferro"=w225:dbl[], "Perdite mecc corrette"=w224:dbl[], "Perdite addiz"=w223:dbl[], "perdite statore corrette"=w222:dbl[], "perdite rotore corrette"=w221:dbl[], "Rendimenti % a carico"=w210:dbl[])
          n147 = Unbundle By Name(w207) -> ("Coeff correlaz"=→"Coeff correlaz":dbl, "Prova da ripetere"=w195:bool)
          n148 = Number To Fractional String(number=w227, precision (6)=w209) -> (F-format string=w220:string[])  [unwired: 2 in]
          n149 = Number To Fractional String(number=w226, precision (6)=w209) -> (F-format string=w219:string[])  [unwired: 2 in]
          n150 = Number To Fractional String(number=w225, precision (6)=w209) -> (F-format string=w218:string[])  [unwired: 2 in]
          n151 = Number To Fractional String(number=w224, precision (6)=w209) -> (F-format string=w217:string[])  [unwired: 2 in]
          n152 = Number To Fractional String(number=w223, precision (6)=w209) -> (F-format string=w216:string[])  [unwired: 2 in]
          n153 = Number To Fractional String(number=w222, precision (6)=w209) -> (F-format string=w215:string[])  [unwired: 2 in]
          n154 = Number To Fractional String(number=w221, precision (6)=w209) -> (F-format string=w214:string[])  [unwired: 2 in]
          n155 = Number To Fractional String(number=w210, precision (6)=w209) -> (F-format string=w208:string[])  [unwired: 2 in]
          n156 = Build Array(w220, w219, w218, w217, w216, w215, w214, w208) -> (w155:string[][])
          n157 = Replace Array Subset(array=w211, new element=w155, index (row)=1, index (col)=2 ("disabled index (col)")) -> (w154:string[][])
          "DETERMINAZIONE DEL RENDIMENTO" <- w154
          n158 = property on="DETERMINAZIONE DEL RENDIMENTO" class="MCListbox (strict)"("ItemNames"=w154) -> ()  [unwired: 2 in, 2 out]
          n159 = Or(x=w195, y=w193) -> (x .or. y?=→"ripeti prova?":bool)
        }
      }
    }
    frame Error {
    }
  }
  "error out" <- w14
